vi "Jog Single Step.vi"(8 "error in (no error)":errorcluster, 10 "Jog Direction":T1, 11 "ThorlabsLabJack in":refnum<class "ThorlabsLabJack.lvclass">) -> (0 "error out":errorcluster, 3 "ThorlabsLabJack out":refnum<class "ThorlabsLabJack.lvclass">)   [LabVIEW 2018, in "ThorlabsLabJack.lvlib" / "ThorlabsLabJack.lvclass"]
doc: "Commands the Axis to jog the specified direction in a single step size."
uses:
  ThorlabsLabJack.lvclass
  LWS_Base/trunk/LabVIEW/PPLs/Configuration/Axis.lvlibp/Custom Controls/Jog Direction.ctl
  LWS_Base/trunk/LabVIEW/PPLs/Configuration/Axis.lvlibp
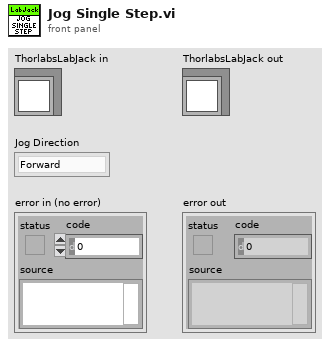
[diagram p1: front panel]
types:
  T1 = typedef "Axis.lvlibp/Jog Direction.ctl" = enum16{"Forward", "Backward"}
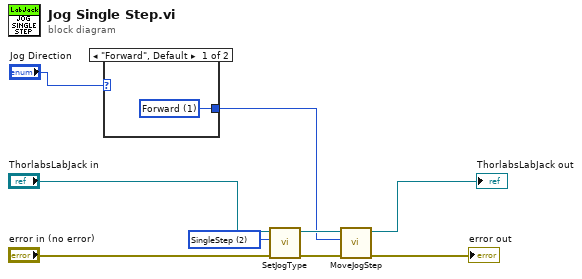
[diagram p0: block diagram]
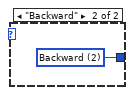
[diagram p2: hidden frame]
diagram:
  w2 = i16 2 items=["ContinuousHeld"=1, "SingleStep"=2, "ContinuousUnheld"=3] ("JogMode")
  n1 = case shown="\"Forward\", Default" "Jog Direction" {
    tunnel: [w10 w11] -> w1
    frame "Forward", Default {
      w10 = 1 items=["Forward"=1, "Backward"=2] ("direction")
    }
    frame "Backward" {
      w11 = 2 items=["Forward"=1, "Backward"=2] ("direction")
    }
  }
  n2 = call "SetJogType.vi"("error in (no error)"="error in (no error)", "JogMode"=w2, "ThorlabsLabJack in"="ThorlabsLabJack in") -> ("error out"=w7:errorcluster, "ThorlabsLabJack out"=w8:refnum<class "ThorlabsLabJack.lvclass">)  [unwired: 7 in]
  n3 = call "MoveJogStep.vi"("error in (no error)"=w7, "direction"=w1, "ThorlabsLabJack in"=w8) -> ("error out"=→"error out":errorcluster, "ThorlabsLabJack out"=→"ThorlabsLabJack out":refnum<class "ThorlabsLabJack.lvclass">)  [unwired: 7 in]
